vi "WiFi Button_Debounce.vi"   [LabVIEW 2014]
uses:
  <vilib>/Aledyne-TSXperts/Arduino Compatible Compiler for LabVIEW/Code Generator/Arduino APIs/Digital/PinDirection.ctl
  <vilib>/Aledyne-TSXperts/Arduino Compatible Compiler for LabVIEW/Arduino Compatible Compiler for LabVIEW.lvlib
  QwaveSys_ESP8266/QwaveSys_ESP8266.lvlib
panel:
  # "Onboard LED (GPIO16) will be ON"
  # "Press FLASH Button (GPIO0)"
types:
  T1 = typedef "Arduino Compatible Compiler for LabVIEW.lvlib/PinDirection.ctl" = enum16{" INPUT", "OUTPUT", " INPUT_PULLUP"}
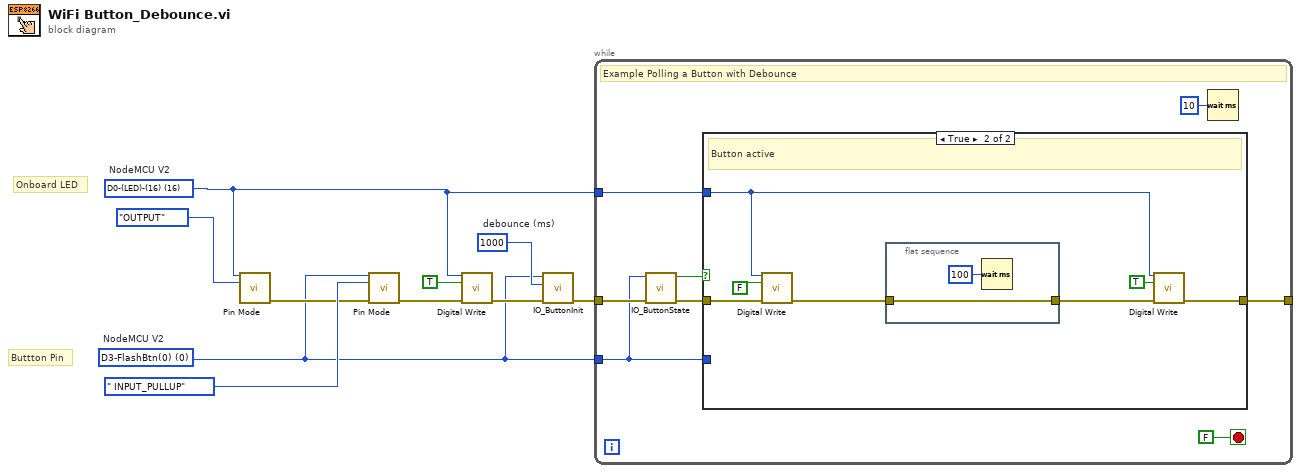
[diagram p0: block diagram]
diagram:
  w1 = u8 0 items=["D0-(LED)-(16)"=16, "D1-SCL(5)"=5, "D2-SDA(4)"=4, "D3-FlashBtn(0)"=0, "D4-(2)"=2, "D5-SCK(14)"=14, "D6-MISO(12)"=12, "D7-MOSI(13)"=13, "D8-SS(15)"=15, "D9-TX(3)"=3, "D10-RX(1)"=1, "ADC0,(17)"=17]  # NodeMCU V2
  w2 = u8 16 items=["D0-(LED)-(16)"=16, "D1-SCL(5)"=5, "D2-SDA(4)"=4, "D3-FlashBtn(0)"=0, "D4-(2)"=2, "D5-SCK(14)"=14, "D6-MISO(12)"=12, "D7-MOSI(13)"=13, "D8-SS(15)"=15, "D9-TX(3)"=3, "D10-RX(1)"=1, "ADC0,(17)"=17]  # NodeMCU V2
  w6 = u16 1000  # debounce (ms)
  # "Buttton Pin"
  # "Onboard LED"
  n1 = call <vilib>:"Pin Mode.vi"("pin"=w2, "direction"=PinDirection."OUTPUT" ("Direction")) -> ("error out"=w5:errorcluster)  [unwired: 13 in]
  n2 = call <vilib>:"Pin Mode.vi"("pin"=w1, "direction"=PinDirection." INPUT_PULLUP" ("Direction"), "error in (no error)"=w5) -> ("error out"=w4:errorcluster)  [unwired: 12 in]
  n3 = call <vilib>:"Digital Write.vi"("pin"=w2, "state"=TRUE, "error in (no error)"=w4) -> ("error out"=w3:errorcluster)  [unwired: 12 in]
  n4 = call "IO_ButtonInit.vi"("error in (no error)"=w3, "debounce (ms)"=w6, "PIN"=w1) -> ("error out"=w7:errorcluster)  [unwired: 8 in]
  n5 = while {
    tunnel: w1 -> [w13]
    tunnel: w2 -> [w16]
    tunnel: [w15] -> _
    tunnel: w7 -> [w14]
    stop <- FALSE stop-if-true
    # "Example Polling a Button with Debounce"
    n6 = call "IO_ButtonState.vi"("error in (no error)"=w14, "PIN"=w13) -> ("error out"=w11:errorcluster, "State"=w12:bool)  [unwired: 8 in]
    n7 = case shown="True" w12 {
      tunnel: w16 -> [_ w26]
      tunnel: w13 -> [_ _]
      tunnel: [w19 w25] -> w15
      tunnel: w11 -> [w19 w24]
      frame False {
        # "Button not active"
      }
      frame True {
        # "Button active"
        n8 = call <vilib>:"Digital Write.vi"("pin"=w26, "state"=FALSE, "error in (no error)"=w24) -> ("error out"=w21:errorcluster)  [unwired: 12 in]
        n9 = flat-sequence {
          tunnel: w21 -> [w28]
          tunnel: [w28] -> w20
          frame #0 {
            n10 = Wait (ms)(milliseconds to wait=u32 100) -> ()  [unwired: 1 out]
          }
        }
        n11 = call <vilib>:"Digital Write.vi"("pin"=w26, "state"=TRUE, "error in (no error)"=w20) -> ("error out"=w25:errorcluster)  [unwired: 12 in]
      }
    }
    n12 = Wait (ms)(milliseconds to wait=u32 10) -> ()  [unwired: 1 out]
  }
